vi "First_Touch_Christmas_Lights.vi"() -> ()   [LabVIEW 2013]
uses:
  Instance           1 21Saved   HandsOn joulu .vi
panel:
  out "Waveform Graph":dynamicdata(graph)
  out "Waveform Chart":dynamicdata(graph)
  in  "Extra contol for blinking\n5 is a good start":dbl
  in  "Blinking frequency":dbl(knob) scale=0.1..0.5
  in  "stop":bool
  out "Valo12":bool
  out "Valo4":bool
  out "Valo11":bool
  out "Valo10":bool
  out "Valo9":bool
  out "Valo8":bool
  out "Valo7":bool
  out "Valo6":bool
  out "Valo5":bool
  out "Valo2":bool
  out "Valo3":bool
  out "Valo1":bool
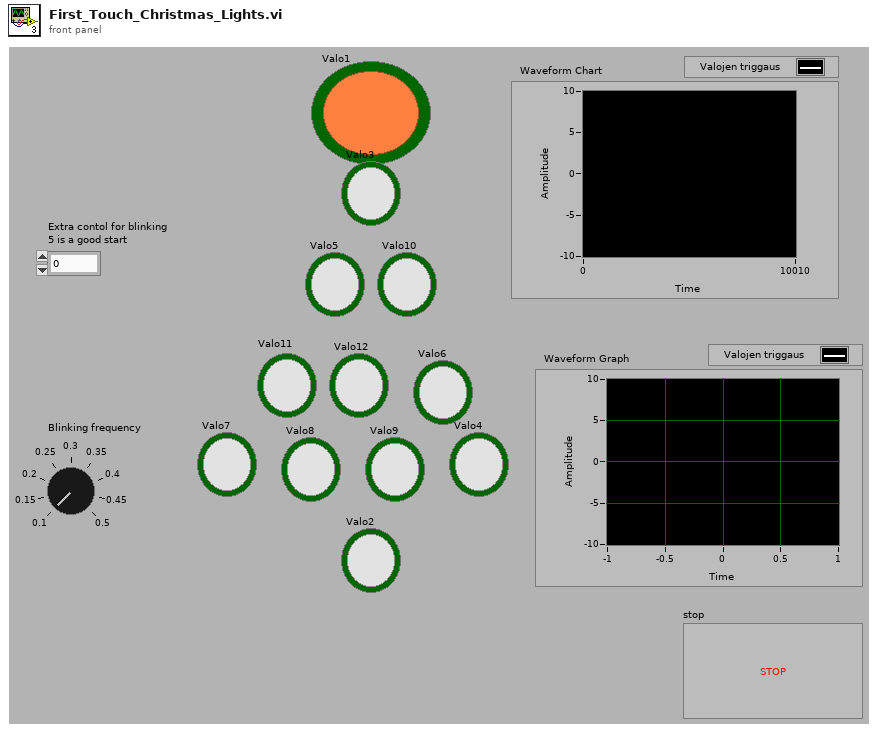
[diagram p1: front panel]
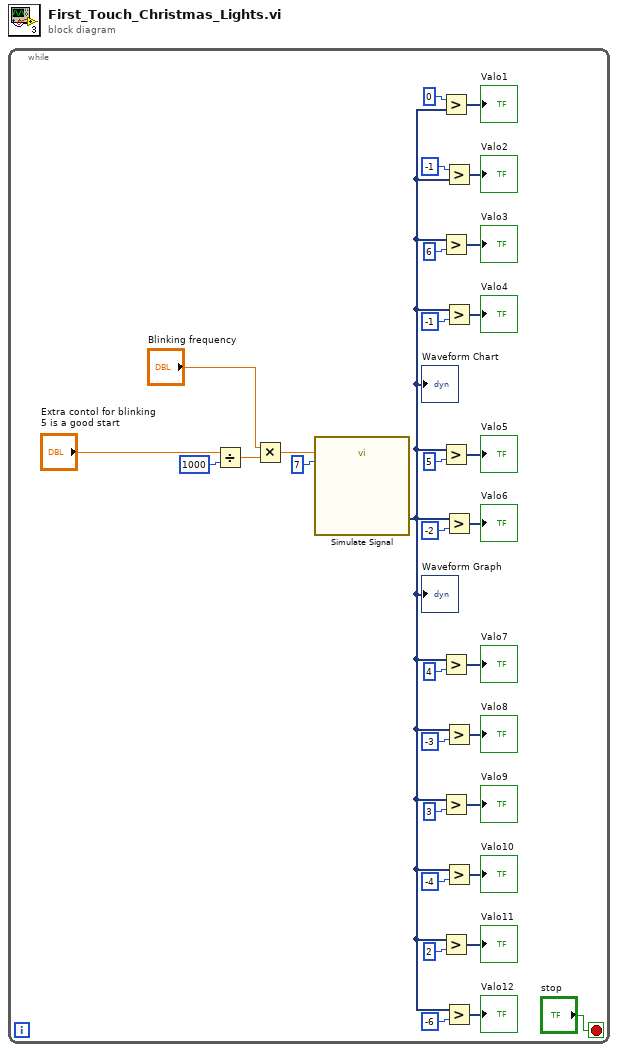
[diagram p0: block diagram]
diagram:
  n1 = while {
    stop <- "stop" stop-if-true
    n2 = Divide(x="Extra contol for blinking\n5 is a good start", y=1000) -> (x/y=w7:dbl)
    n3 = Multiply(x="Blinking frequency", y=w7) -> (x*y=w10:dbl)
    n4 = call "Simulate Signal"("Frequency"=w10, "Amplitude"=7) -> ("Valojen triggaus"=w2:dynamicdata)  [unwired: 12 in, 1 out]
    "Waveform Chart" <- w2
    "Waveform Graph" <- w2
    n5 = Greater?(x=0, y=w2) -> (0:→"Valo1":dynamicdata)
    n6 = Greater?(x=w2, y=6) -> (0:→"Valo3":dynamicdata)
    n7 = Greater?(x=w2, y=5) -> (0:→"Valo5":dynamicdata)
    n8 = Greater?(x=w2, y=4) -> (0:→"Valo7":dynamicdata)
    n9 = Greater?(x=w2, y=3) -> (0:→"Valo9":dynamicdata)
    n10 = Greater?(x=w2, y=2) -> (0:→"Valo11":dynamicdata)
    n11 = Greater?(x=-1, y=w2) -> (0:→"Valo2":dynamicdata)
    n12 = Greater?(x=w2, y=-1) -> (0:→"Valo4":dynamicdata)
    n13 = Greater?(x=w2, y=-2) -> (0:→"Valo6":dynamicdata)
    n14 = Greater?(x=w2, y=-3) -> (0:→"Valo8":dynamicdata)
    n15 = Greater?(x=w2, y=-4) -> (0:→"Valo10":dynamicdata)
    n16 = Greater?(x=w2, y=-6) -> (0:→"Valo12":dynamicdata)
  }
